vi "GetCaseFrameNamesWhereInVI.vi"(11 "reference":refnum<vi>) -> (3 "FrameNames":string[](array[string]))   [LabVIEW 2015]
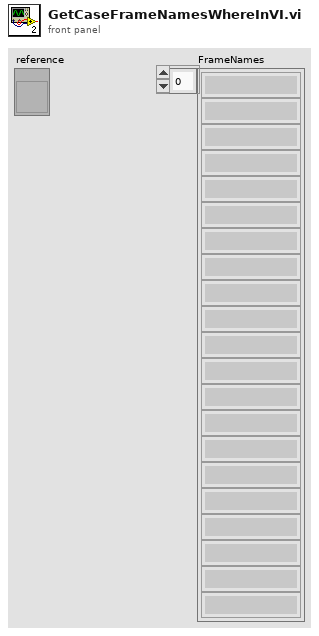
[diagram p1: front panel]
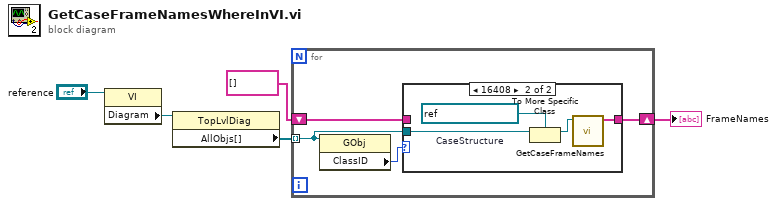
[diagram p0: block diagram]
diagram:
  n1 = property class="VI"(reference="reference") -> ("Diagram"=w5:refnum<vi>)  [unwired: 1 in, 2 out]
  n2 = property class="TopLvlDiag"(reference=w5) -> ("AllObjs[]"=w4:refnum<vi>[])  [unwired: 1 in, 2 out]
  n3 = for {
    tunnel: w4 -> [w8] mode=indexing
    shift-right: [w7] -> w2
    shift-left: string[] [] ("FrameNames") -> [w6]
    n4 = property class="GObj"(reference=w8) -> ("ClassID"=w9:u32)  [unwired: 1 in, 2 out]
    n5 = case shown="16408" w9 {
      tunnel: w8 -> [_ w14]
      tunnel: [w10 w11] -> w7
      tunnel: w6 -> [w10 _]
      frame Default {
      }
      frame 16408 {
        w13 = refnum<vi> refnum  # CaseStructure
        n6 = To More Specific Class(target class=w13, reference=w14) -> (specific class reference=w12:refnum<vi>)  [unwired: 1 in, 1 out]
        n7 = call "GetCaseFrameNames.vi"("Case reference"=w12) -> ("FrameNames"=w11:string[])  [unwired: 10 in]
      }
    }
  }
  "FrameNames" <- w2
